vi "Temperature Warnings.vi"(8 "Error In":errorcluster, 11 "Weather Data In":T1={"Current Temperature"=0.0, "Max Temperature"=0.0, "Min Temperature"=0.0, "Warning?"=FALSE, "Warning Text"="No Warning", "Units"=enum."Celcius", "Current Windspeed"=0.0, "Max Windspeed"=0.0, "Windspeed Warning?"=FALSE, "Windspeed Warning Text"="No Warning"}) -> (0 "Error Out":errorcluster, 3 "Weather Data 2 Out":T1={"Current Temperature"=0.0, "Max Temperature"=0.0, "Min Temperature"=0.0, "Warning?"=FALSE, "Warning Text"="No Warning", "Units"=enum."Celcius", "Current Windspeed"=0.0, "Max Windspeed"=0.0, "Windspeed Warning?"=FALSE, "Windspeed Warning Text"="No Warning"})   [LabVIEW 2017]
doc: "This VI is used to determine the string to output to the weather station based on the current temperature and limit settings.\n\nInputs: Current Temperature (DBL), Minimum Temperature (DBL), and Maximum Temperature (DBL).\nOutputs: Warning Text (string) and Warning? (Boolean)."
uses:
  Weather Data.ctl
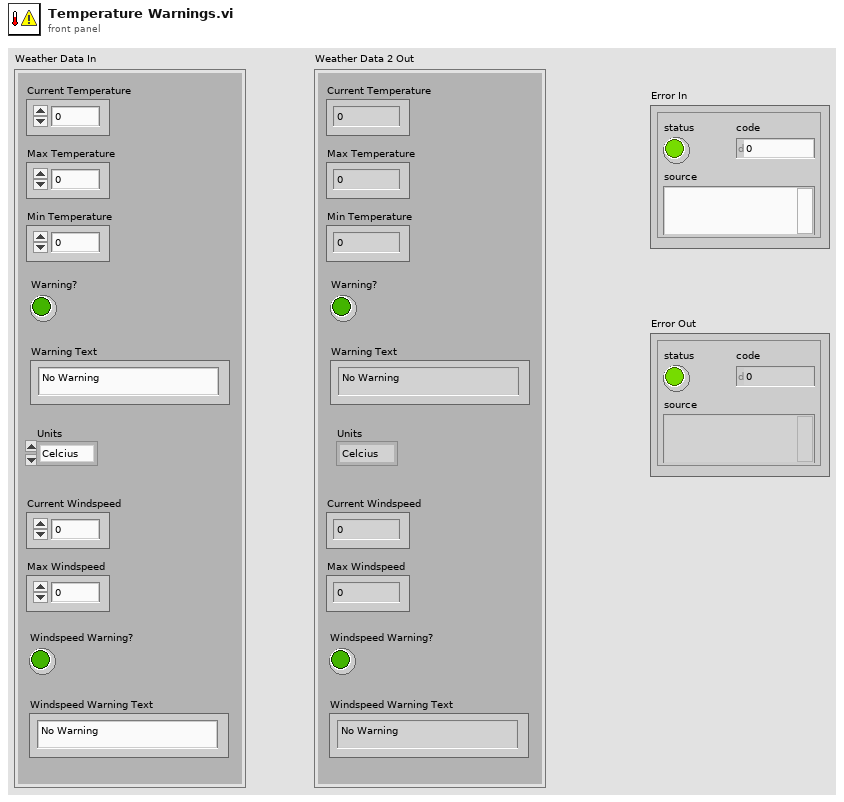
[diagram p1: front panel]
types:
  T1 = typedef "Weather Data.ctl" = cluster{"Current Temperature":dbl, "Max Temperature":dbl, "Min Temperature":dbl, "Warning?":bool, "Warning Text":string, "Units":enum16{"Celcius", "Farenheit"}, "Current Windspeed":dbl, "Max Windspeed":dbl, "Windspeed Warning?":bool, "Windspeed Warning Text":string}
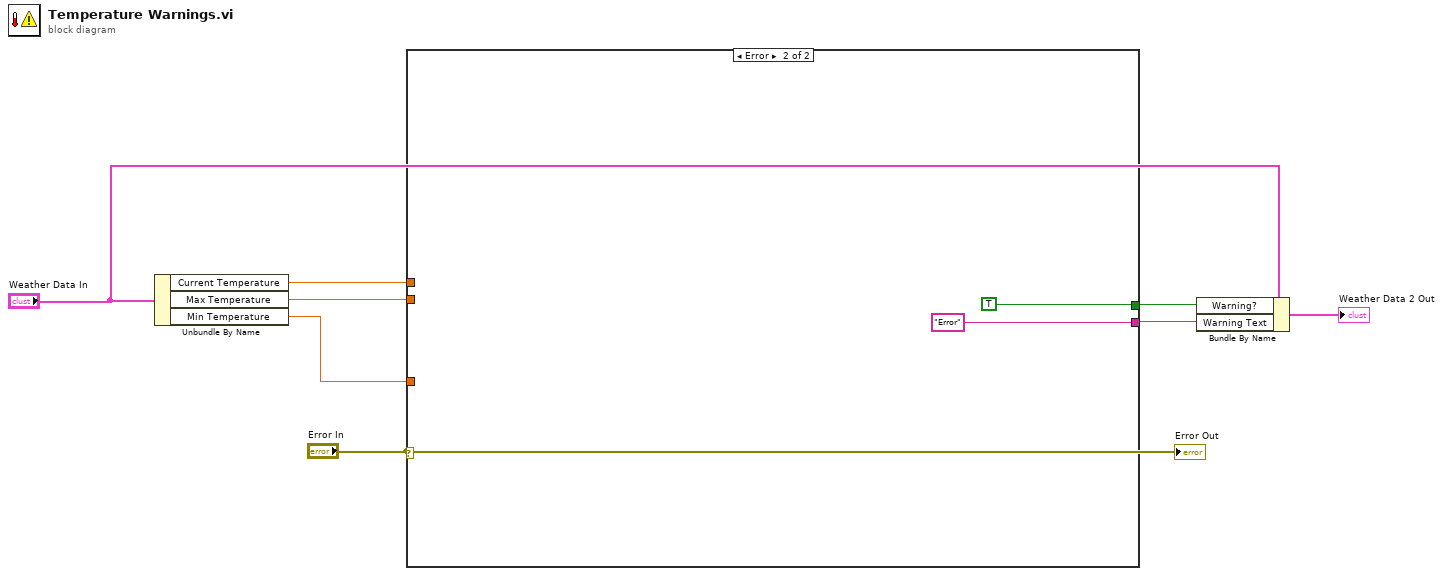
[diagram p0: block diagram]
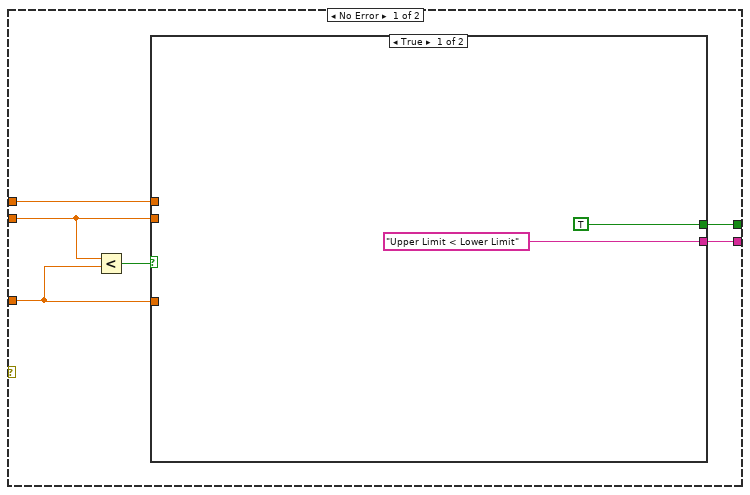
[diagram p2: hidden frame]
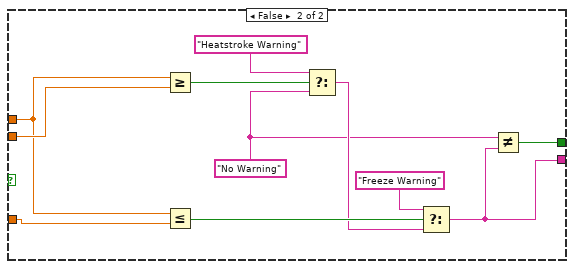
[diagram p3: hidden frame]
diagram:
  n1 = Unbundle By Name("Weather Data In") -> ("Current Temperature"=w7:dbl, "Max Temperature"=w8:dbl, "Min Temperature"=w6:dbl)
  n2 = case shown="Error" "Error In" {
    tunnel: w8 -> [w12 _]
    tunnel: w7 -> [w14 _]
    tunnel: w6 -> [w11 _]
    tunnel: [w10 TRUE] -> w3
    tunnel: [w13 "Error"] -> w2
    frame No Error {
      n3 = Less?(x=w12, y=w11) -> (x < y?=w9:bool)
      n4 = case shown="True" w9 {
        tunnel: w12 -> [_ w21]
        tunnel: w14 -> [_ w20]
        tunnel: w11 -> [_ w19]
        tunnel: ["Upper Limit < Lower Limit" w17] -> w13
        tunnel: [TRUE w18] -> w10
        frame True {
        }
        frame False {
          w22 = "No Warning" ("f")
          n5 = Greater Or Equal?(x=w20, y=w21) -> (x >= y?=w27:bool)
          n6 = Less Or Equal?(x=w20, y=w19) -> (x <= y?=w24:bool)
          n7 = Select(t="Heatstroke Warning", s=w27, f=w22) -> (s? t:f=w23:string)
          n8 = Select(t="Freeze Warning", s=w24, f=w23) -> (s? t:f=w17:string)
          n9 = Not Equal?(x=w22, y=w17) -> (x != y?=w18:bool)
        }
      }
    }
    frame Error {
    }
  }
  n10 = Bundle By Name(cluster="Weather Data In", "Warning?"=w3, "Warning Text"=w2) -> (→"Weather Data 2 Out":T1)
  "Error Out" <- "Error In"
